vi "CreateTriggerNode.vi"(7 "DOM Document":refnum<k20>, 8 "Error In":errorcluster, 11 "Trigger Configuration":T1={"Arm"={"Source"=enum."Hold", "Count"=1, "Infinite?"=FALSE}, "Scan"={"Source"=enum."Hold", "Count"=0, "Infinite?"=FALSE, "Delay (sec)"=0.0, "Interval (sec)"=0.0}, "Channel"={"Source"=enum."Hold", "Count"=0, "Infinite?"=FALSE, "Auto Count?"=FALSE, "Delay (sec)"=0.0, "Interval (sec)"=0.0}} {"Arm"."Count" min=1 max=99999 step=1}) -> (0 "Error Out":errorcluster, 3 "Trigger Node":refnum<k20>)   [LabVIEW 2012]
uses:
  TriggerConfiguration.ctl
  TriggerArmConfiguration.ctl
  driver/Public/Controls/ArmSource.ctl
  TriggerScanConfiguration.ctl
  driver/Public/Controls/ScanSource.ctl
  TriggerChannelConfiguration.ctl
  driver/Public/Controls/TriggerSource.ctl
  libs/LV-Utilities/LV-Utilities.lvlib
  driver/Keithley-7001.lvlib
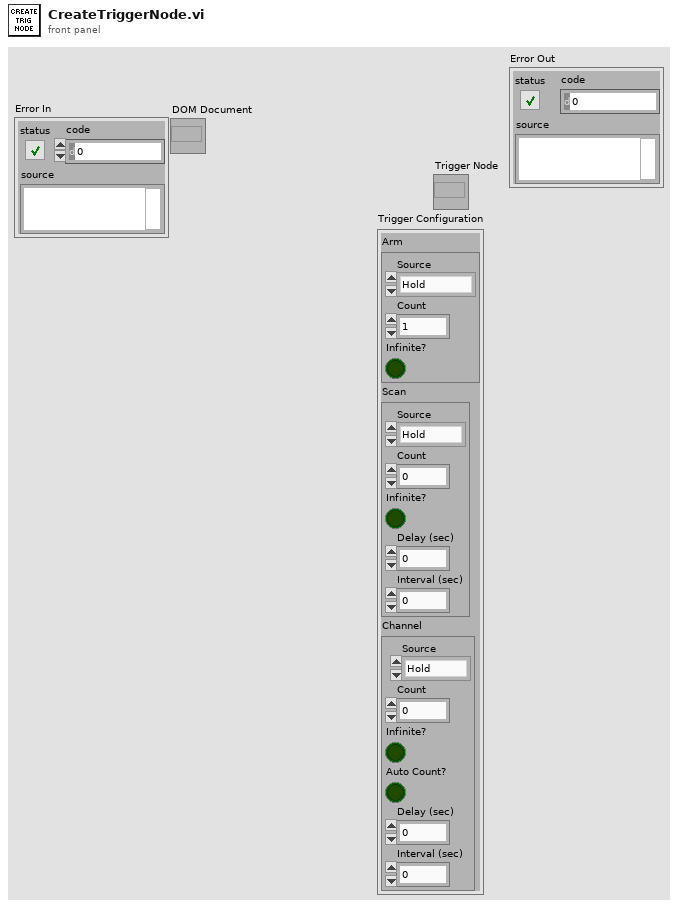
[diagram p1: front panel]
types:
  T1 = typedef "TriggerConfiguration.ctl" = cluster{"Arm":T2, "Scan":T4, "Channel":T6}
  T2 = typedef "TriggerArmConfiguration.ctl" = cluster{"Source":T3, "Count":u32, "Infinite?":bool}
  T3 = typedef "Keithley-7001.lvlib/ArmSource.ctl" = enum16{"Hold", "Immediate", "Manual", "Bus", "TLink", "External"}
  T4 = typedef "TriggerScanConfiguration.ctl" = cluster{"Source":T5, "Count":u32, "Infinite?":bool, "Delay (sec)":dbl, "Interval (sec)":dbl}
  T5 = typedef "Keithley-7001.lvlib/ScanSource.ctl" = enum16{"Hold", "Immediate", "Timer", "Manual", "Bus", "TLink", "External"}
  T6 = typedef "TriggerChannelConfiguration.ctl" = cluster{"Source":T7, "Count":u32, "Infinite?":bool, "Auto Count?":bool, "Delay (sec)":dbl, "Interval (sec)":dbl}
  T7 = typedef "Keithley-7001.lvlib/TriggerSource.ctl" = enum16{"Hold", "Immediate", "Manual", "Bus", "TLink", "External", "Timer"}
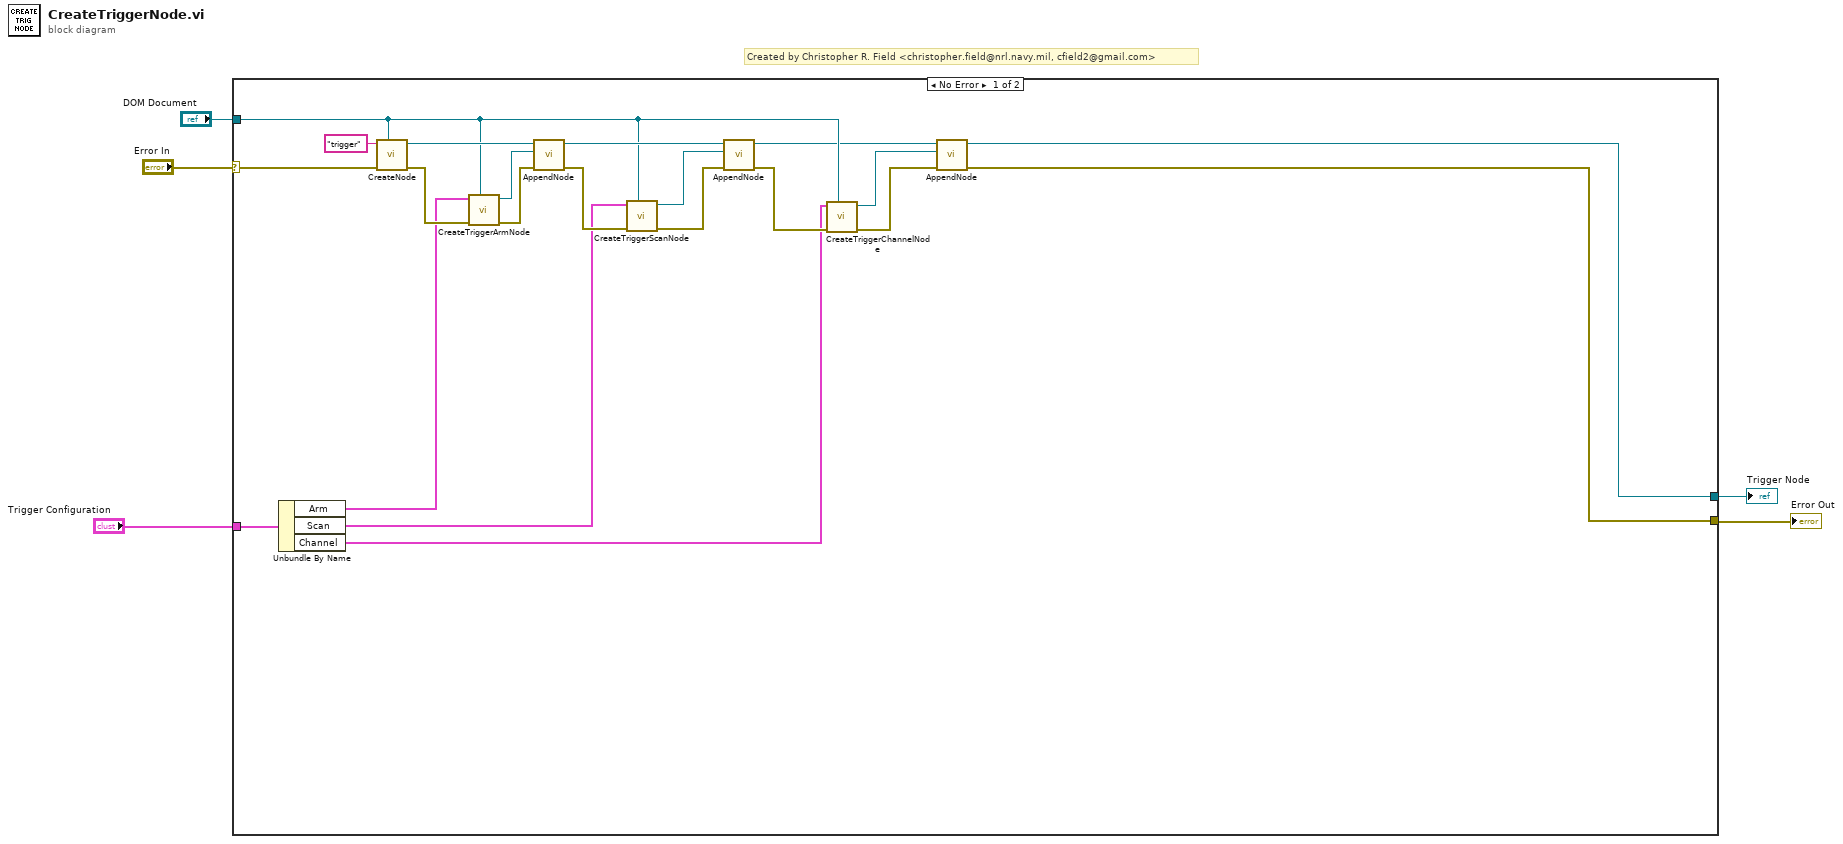
[diagram p0: block diagram]
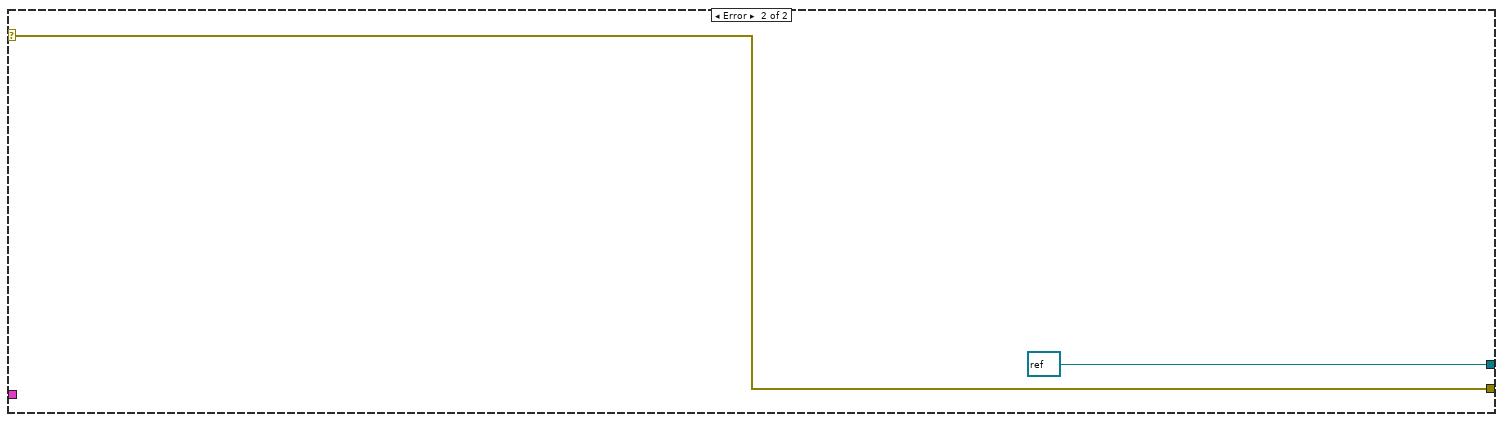
[diagram p2: hidden frame]
diagram:
  # "Created by Christopher R. Field <christopher.field@nrl.navy.mil, cfield2@gmail.com>"
  n1 = case shown="No Error" "Error In" {
    selector: "Error In" -> [w26 w28]
    tunnel: "DOM Document" -> [w11 _]
    tunnel: [w23 w28] -> w3
    tunnel: [w24 refnum<k20> refnum ("Wirings Node 2")] -> w2
    tunnel: "Trigger Configuration" -> [w22 _]
    frame No Error {
      n2 = Unbundle By Name(w22) -> ("Arm"=w20:T2, "Scan"=w15:T4, "Channel"=w6:T6)
      n3 = call "CreateNode.vi"("DOM Document"=w11, "Error In"=w26, "Tag Name"="trigger") -> ("Error out"=w21:errorcluster, "Node"=w19:refnum<k20>)  [unwired: 7 in]
      n4 = call "CreateTriggerArmNode.vi"("DOM Document"=w11, "Error In"=w21, "Trigger Arm Configuration"=w20) -> ("Error Out"=w17:errorcluster, "Trigger Arm Node"=w18:refnum<k20>)  [unwired: 7 in]
      n5 = call "AppendNode.vi"("Error In"=w17, "Child Node"=w18, "Parent Node In"=w19) -> ("Error Out"=w16:errorcluster, "Parent Node Out"=w14:refnum<k20>)  [unwired: 7 in]
      n6 = call "CreateTriggerScanNode.vi"("DOM Document"=w11, "Error In"=w16, "Trigger Scan Configuration"=w15) -> ("Error Out"=w12:errorcluster, "Trigger Scan Node"=w13:refnum<k20>)  [unwired: 7 in]
      n7 = call "AppendNode.vi"("Error In"=w12, "Child Node"=w13, "Parent Node In"=w14) -> ("Error Out"=w10:errorcluster, "Parent Node Out"=w9:refnum<k20>)  [unwired: 7 in]
      n8 = call "CreateTriggerChannelNode.vi"("DOM Document"=w11, "Error In"=w10, "Trigger Channel Configuration"=w6) -> ("Error Out"=w7:errorcluster, "Trigger Channel Node"=w8:refnum<k20>)  [unwired: 7 in]
      n9 = call "AppendNode.vi"("Error In"=w7, "Child Node"=w8, "Parent Node In"=w9) -> ("Error Out"=w23:errorcluster, "Parent Node Out"=w24:refnum<k20>)  [unwired: 7 in]
    }
    frame Error {
    }
  }
  "Trigger Node" <- w2
  "Error Out" <- w3
